vi "Read Water Level Actor.vi"(11 "仿真冷却器":refnum<class "Simulated Evaporative Cooler.lvclass">) -> (2 "水位":refnum<class "Water Level.lvclass">)   [LabVIEW 2013, in "Simulated Evaporative Cooler.lvclass"]
uses:
  Simulated Evaporative Cooler.lvclass
  Water Level/Water Level.lvclass
  Simulated Water Level/Simulated Water Level.lvclass
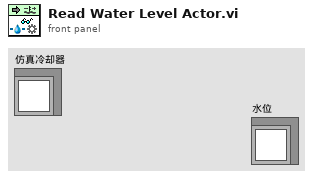
[diagram p1: front panel]
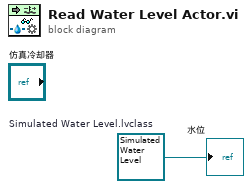
[diagram p0: block diagram]
diagram:
  w1 = refnum<class "Simulated Water Level.lvclass"> refnum  # Simulated Water Level.lvclass
  "水位" <- w1
